vi "Main.vi"() -> ()   [LabVIEW 2012]
uses:
  ChannelStateControl.ctl
  <vilib>/Utility/error.llb/DialogType.ctl
  Imaging Pulse Control/Examples/Support/Channel Parameters.ctl
  Imaging Pulse Control/Examples/Support/System Parameters.ctl
  <vilib>/UeiDaq/UeiDaqCreateDOSession.vi
  <vilib>/UeiDaq/UeiDaqConfigureTimingForSimpleIO.vi
  <vilib>/ULx/Create Channel.llb/ULx Create Channel (AO-Voltage-Basic).vi
  <vilib>/ULx/Write.llb/ULx Write (Analog 1D DBL NChan 1Samp).vi
  <vilib>/UeiDaq/UeiDaqWriteDigitalDataUInt16.vi
  <vilib>/UeiDaq/UeiDaqWriteOneDigitalScanUInt16.vi
  <resource>/objmgr/UeiDaq.rc
  Imaging Pulse Control/Quantum Composers 9000 Series.lvlib
  IPG Pulse Control/Agilent 33XXX Series.lvlib
  Agilent ESG Series/Agilent ESG Series.lvlib
panel:
  in  "Composer Write":bool
  in  "VISA session":refnum<visa-resource-name>
  in  "error in (no error)":errorcluster {"code" format="%.0x"}
  out "error out":errorcluster {"code" format="%.0x"}
  in  "Frequency (MHz)":dbl=224.0 format="%.11f"
  in  "Amplitude (dBm)":dbl=7.0 format="%.2f"
  in  "Output Enable":bool=TRUE
  out "Offset":dbl
  out "Amplitude":dbl
  in  "Maximum Voltage":dbl=10.0
  in  "Initial Voltage":dbl=2.0
  in  "Final Voltage":dbl=4.0
  out "Frequency":dbl=0.4838
  in  "Trigger Source (0: Internal)":u16(ring)=1 items=["Internal", "External", "Software (bus)"]
  in  "Enable Burst":bool=TRUE
  in  "Burst Mode (0: Triggered)":u16(ring) items=["Triggered", "Gated"]
  out "Simulated WaveForm":dbl[](graph)
  out "Total Time  (<16000)":i32
  in  "Final Keep Time":i32=100
  in  "Fall Down Time":i32=1000
  in  "Rise Up Time":i32=15
  in  "Pulse Width":i32=100
  in  "Inintial Voltage Time":i32=1
  in  "IPG Controller (Agilent 33210A)":refnum<visa-resource-name>
  in  "Arbitrary Waveform Name":string="ARB1"
  in  "Run IPG Laser Control":bool
  in  "Normal Stop":bool
  in  "Voltage (V)":dbl[](array[numeric])
  in  "Initial States(Adjustable)":u16[](array[numeric])=[0, 0, 0, 0, 0, 0, 0, 0, 0, 0, 0, 0, 0, 0, 0, 0, 0, 0, 0, 0] caption="Initial States"
  in  "DIO Groups":T1[](array[typedef])
  out "Quantum Composer Command":string[](array[string])
  in  "Sys Period (s)":dbl=0.15
  out "Composer Ready?":bool
  out "Main Loop Stopped?":bool
  in  "Quantum Composer Resource":refnum<visa-resource-name>
  in  "Run/Stop":bool caption="stop"
  in  "Exit":bool
  out "Running 2":bool
  in  "Maximum Value":dbl=5.5 format="%0.2f"
  in  "Minimum Value":dbl format="%0.2f"
  out "Status Indicator":bool[][](array[boolean])
  out "Total Step":u64
  in  "Original Timing Signal (adjustable)":i16[][](array[numeric])=[[0, 0, 0, 0, 0, 0, 0, 0, 0, 0, 0, 0, 0, 0, 0, 0, 0, 0, 0, 0]] format="%b"
  out "Running":bool
  in  "DIO Port":string="pwrdaq://Dev0/Do0:2"
  in  "stop":bool
  out "Loop Count":i32
  in  "Loop":bool
  out "Parsed File Location":path
  in  "All Low":bool
  in  "Run":bool
  in  "Timing Array (Adjustable)":i32[](array[numeric])=[0, 0, 0, 0, 0, 0, 0, 0, 0, 0, 0, 0, 0, 0, 0, 0, 0, 0, 0, 0] caption="Timing Array (Time Duration for each signal)"
  out "Modified Timing Signal":u16[][](array[numeric]) caption="Modified Timing Signal (after adjustment from I/O channel panel)" format="%b"
  in  "Compile":bool
  out "Channel Names":string[](array[string])
  in  "Channel Number (Adjustable)":u16=48
  in  "Load":bool
  in  "Timing File":path
  in  "Perl Parser":path=path "C:/Labview/Parser File/parse-timing.pl"
  # "MCCDAQ Control"
  # "(Use Do0:5 for DIO0-DIO5, 6ch,  Do0;5 for DIO0 and DIO5, 2ch)"
  # "Control Panel"
  # "(pwrdaq://Dev0 for real I/O; simu://Dev2 for simulated DAQ card)"
  # "1"
  # "2"
  # "3"
  # "4"
  # "5"
  # "6"
  # "7"
  # "8"
  # "9"
  # "10"
  # "11"
  # "12"
  # "13"
  # "14"
  # "15"
  # "16"
  # "Quantum Composer Control"
  # "Read me: (Very Important!!!!!!!!!)\n1. This Labview is used to control the IPG laser output power, When you edit this programme make sure the IPG laser is off.\n2. follow the steps, First is the visa address setting; Second is the pulse edit; Third is the output checking; Forth is the trigger set .\n3. The maximum input voltage is 10V, the minmum value is 1V. The total input time must smaller than 16000ms and larger than 8 ms."
  # "Group1"
  # "Group2"
  # "Group3"
  # "IPG Modulation Control"
  # "Offset Locking Control"
  # "Group4"
  # "Group5"
  # "Group6"
  # "(Currently, When \"STOP Loop\" is pressed, the status remain in the final state, when Stop Program or ER stop is pressed, all channels will be set as \"low\")"
  # "Status Panel"
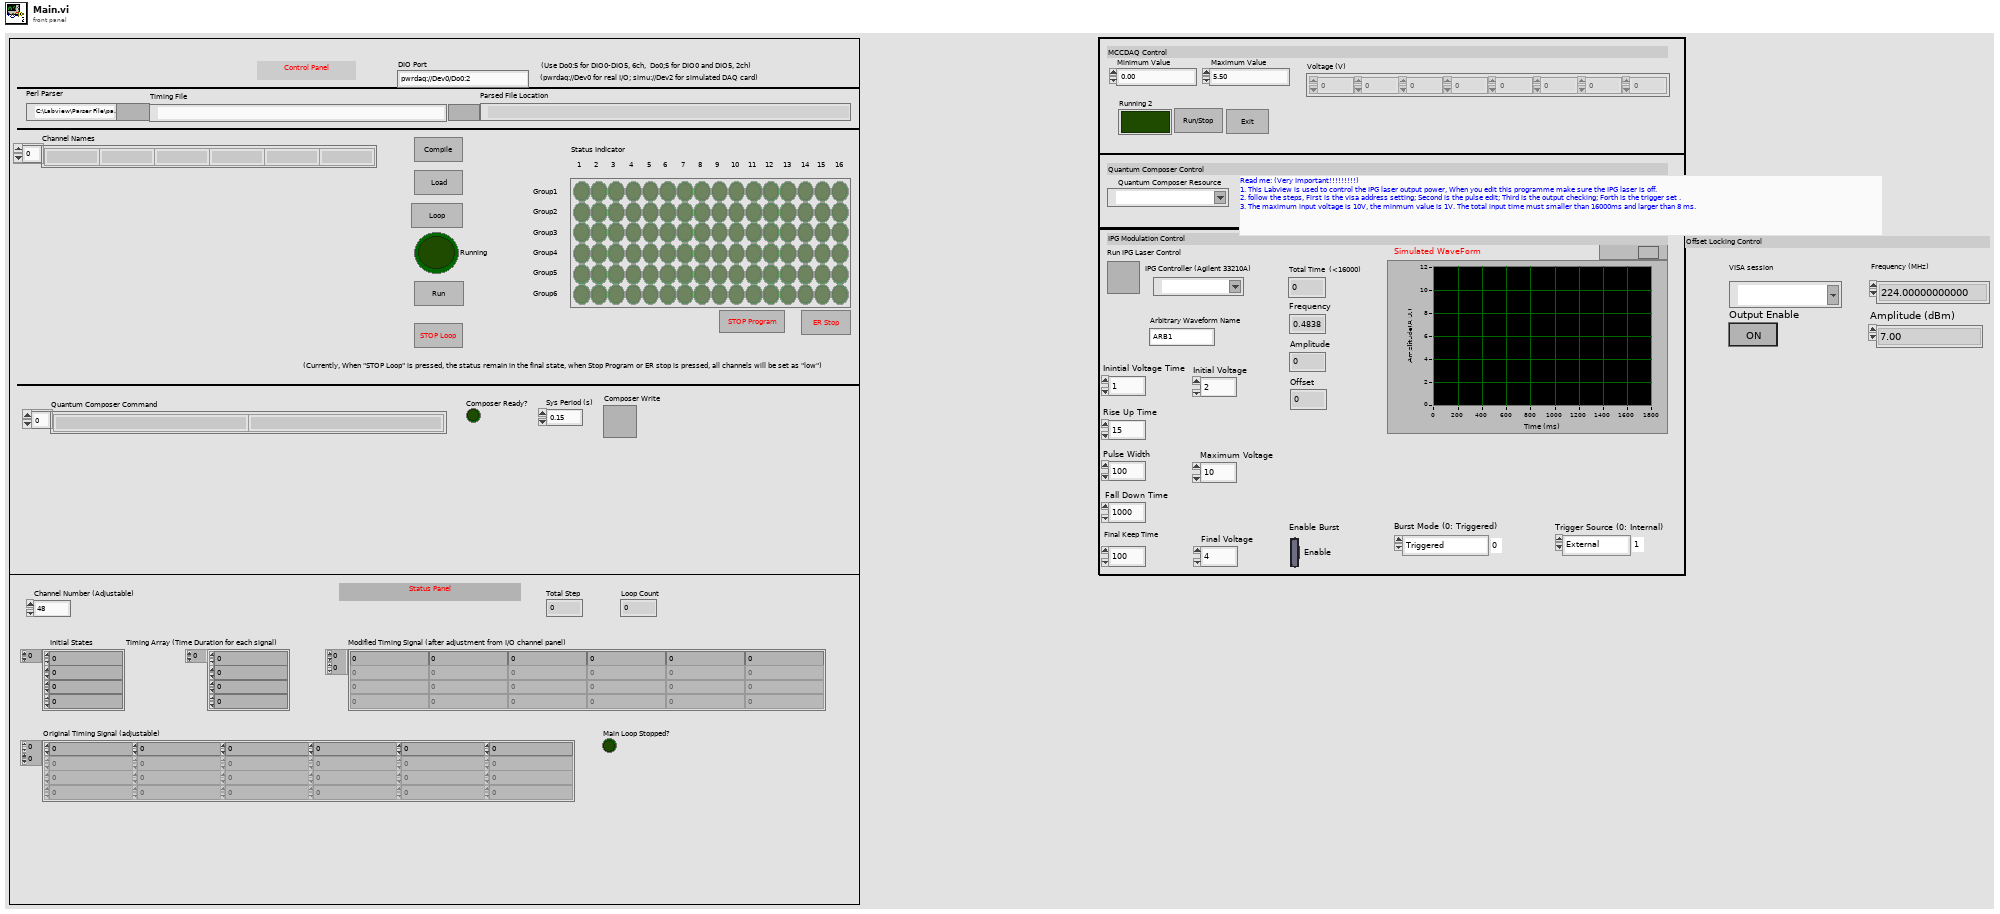
[diagram p1: front panel]
types:
  T1 = typedef "ChannelStateControl.ctl" = cluster{"Channel 1":u8, "Enable":bool, "Main Switch":u8, "Channel 2":u8, "Channel 9":u8, "Channel 10":u8, "Channel 11":u8, "Channel 3":u8, "Channel 4":u8, "Channel 12":u8, "Channel 5":u8, "Channel 13":u8, "Channel 6":u8, "Channel 14":u8, "Channel 7":u8, "Channel 15":u8, "Channel 8":u8, "Channel 16":u8}
  T2 = typedef "Channel Parameters.ctl" = cluster{"Channel":i32, "Chan State":bool, "Chan Sync Source":i32, "Chan Gate Logic":enum16{"Disabled", "Low", "High"}, "Chan Mode":enum16{"Normal", "Single", "Burst", "Duty Cycle"}, "Chan Wait #":i32, "Chan Delay":dbl, "Chan Width":dbl, "Chan Burst #":i32, "Chan DC On":i32, "Chan DC Off":i32, "Chan Polarity":bool, "Chan MUX Value":i32, "Chan Level Out":enum16{"TTL", "Adjustable", "35 Volt", "Optical"}, "Chan Lev Adjust":dbl, "Chan Gate Mode":enum16{"Disabled", "Pulse Inhibit", "Output Inhibit"}}
  T3 = typedef "DialogType.ctl" = u16
  T4 = typedef "System Parameters.ctl" = cluster{"Sys Period":dbl, "Sys Mode":enum16{"Normal", "Single", "Burst", "Duty Cycle"}, "Sys Burst #":i32, "Sys DC On":i32, "Sys DC Off":i32, "Sys State":bool, "Sys Gate":bool, "Sys Trig Edge":bool, "Sys Ext Mode":enum16{"Disabled", "Triggered", "Gated", "Triggered & Gated"}, "Sys Trig Lev":dbl, "Sys Gate Lev ":dbl, "Sys Gate Mode":enum16{"Disabled", "Pulse Inhibit", "Output Inhibit", "Channel"}}
  T5 = cluster{"Baud Rate":u32, "Parity":u16, "Data Bits":u16, "Flow Control":u16}
  T6 = enum16{"dBm", "dBuV", "dBuVemf", "mV", "uV", "mVemf", "uVemf"}
  T7 = enum16{"SINE", "TRIANGLE", "SQUARE", "RAMP", "NOISE", "DUAL SINE", "SWEPT SINE"}
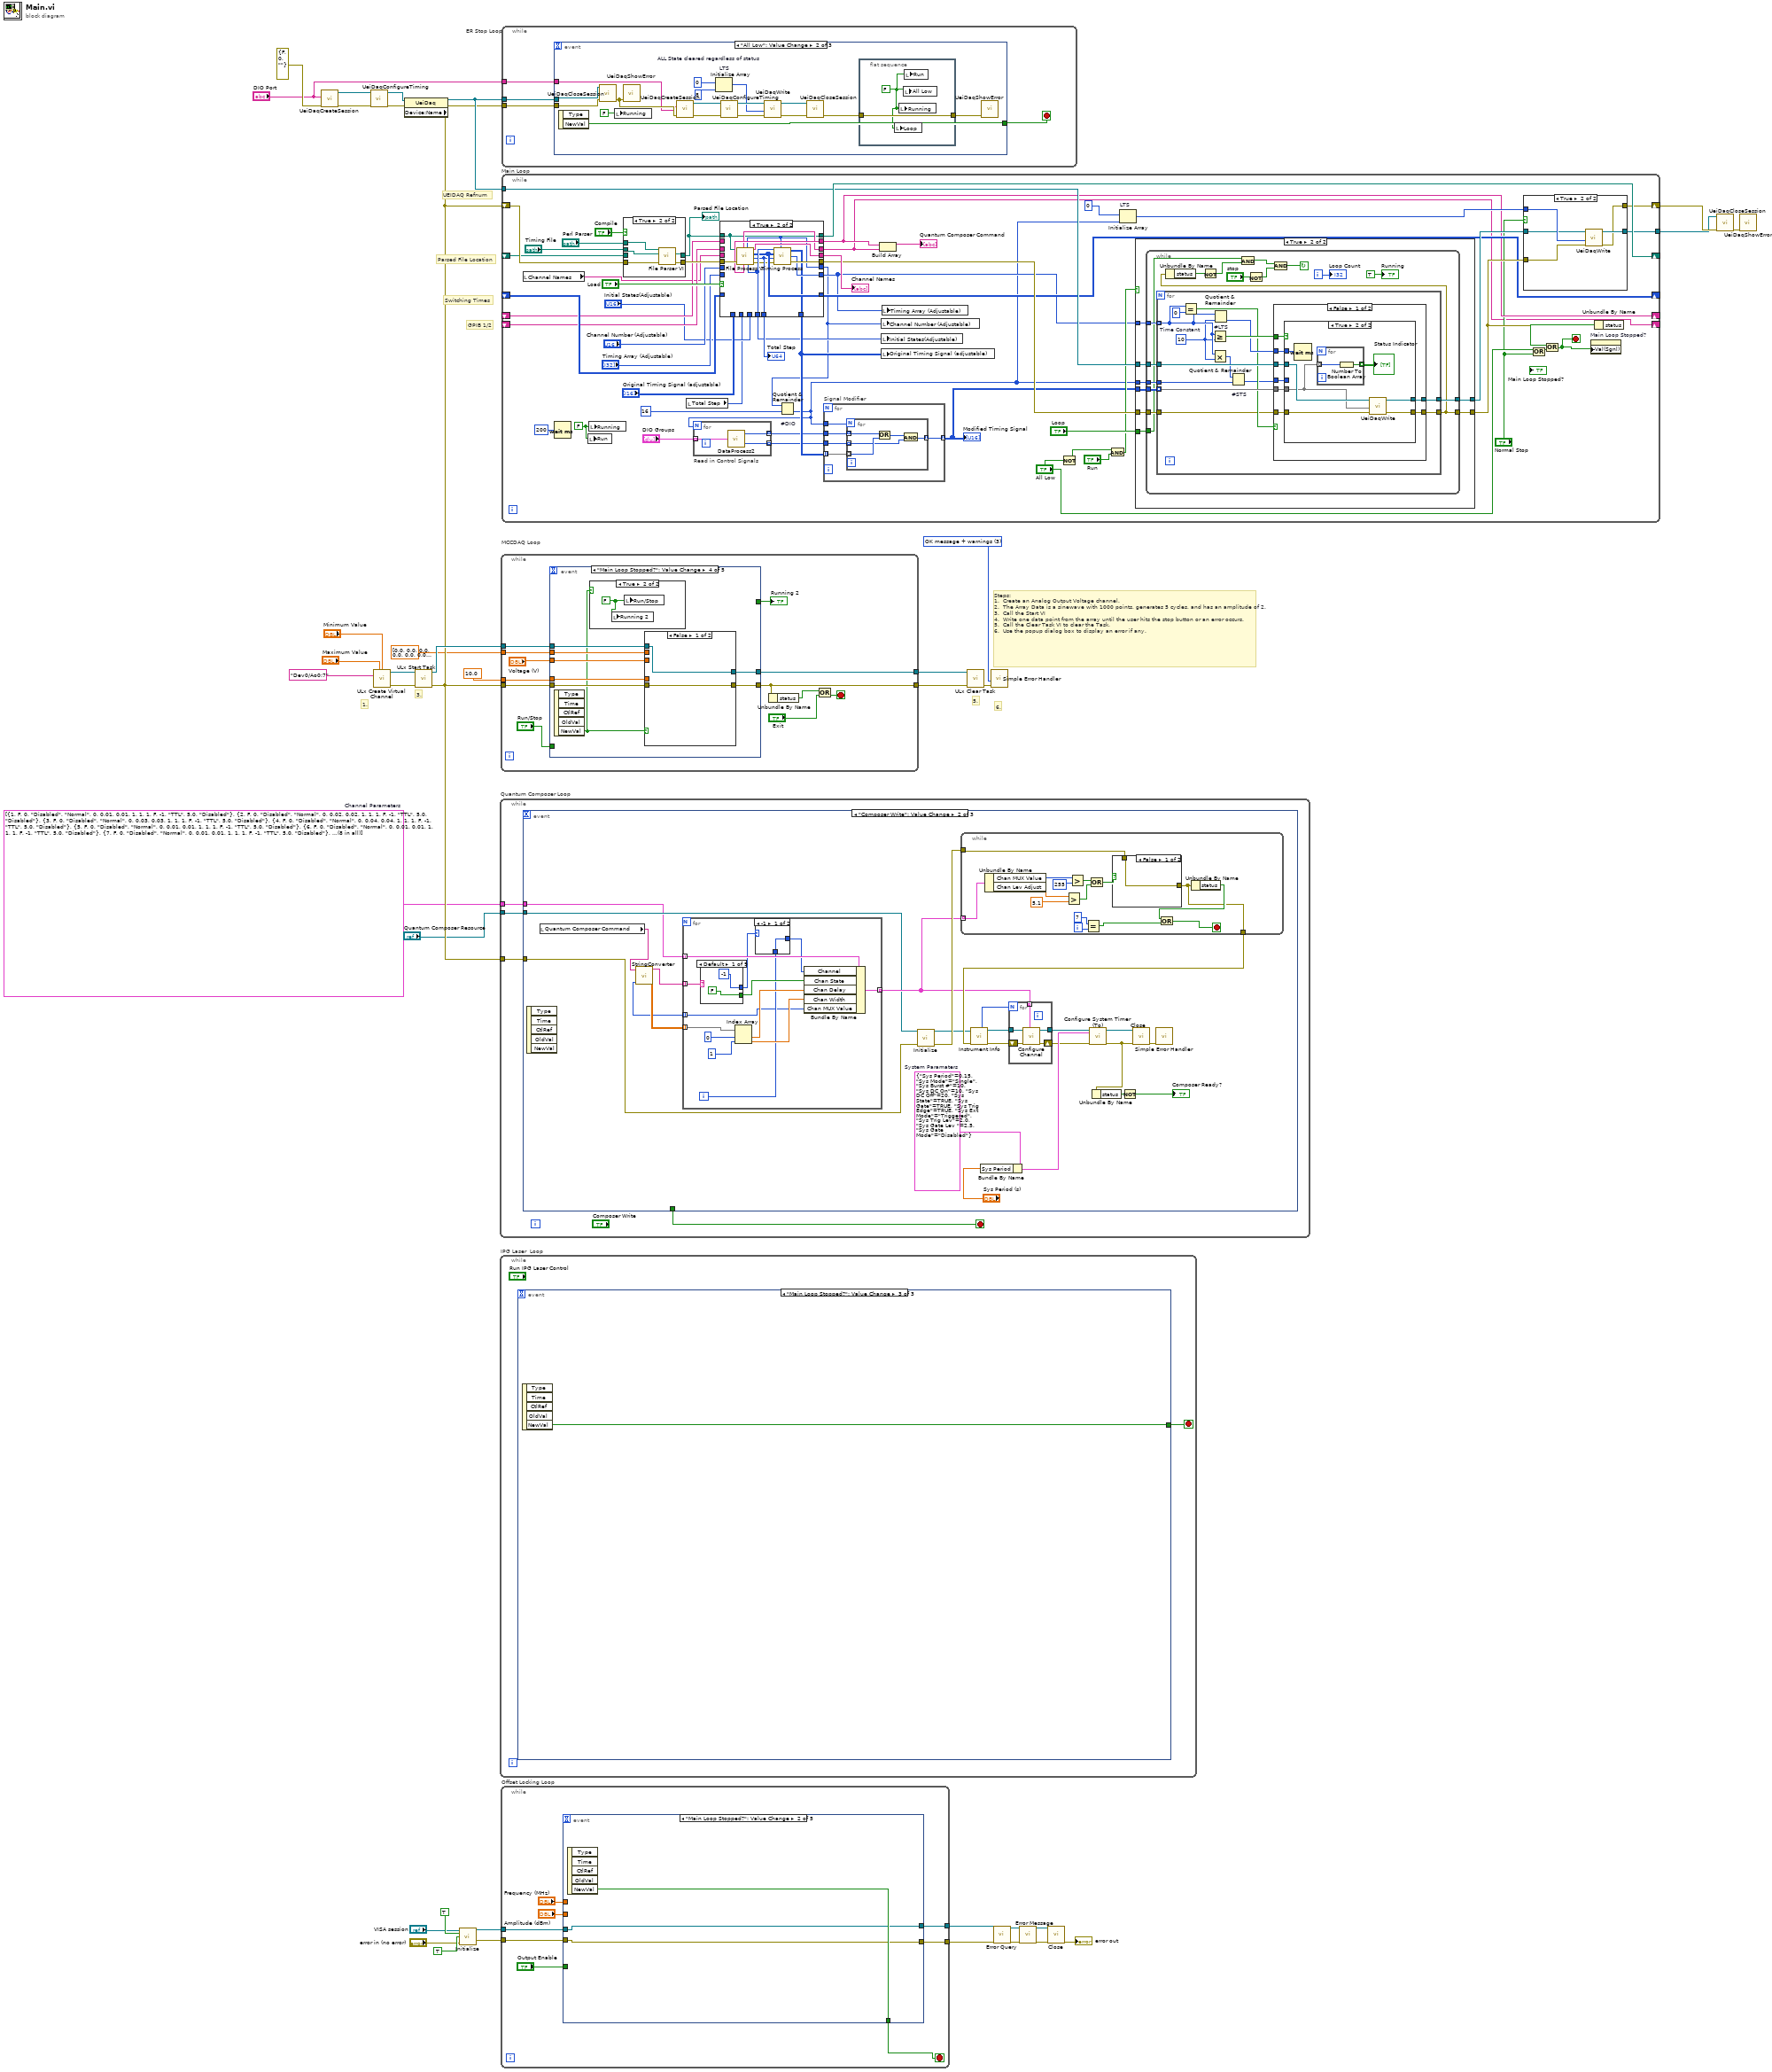
[diagram p0: block diagram]
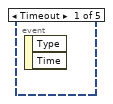
[diagram p2: hidden frame]
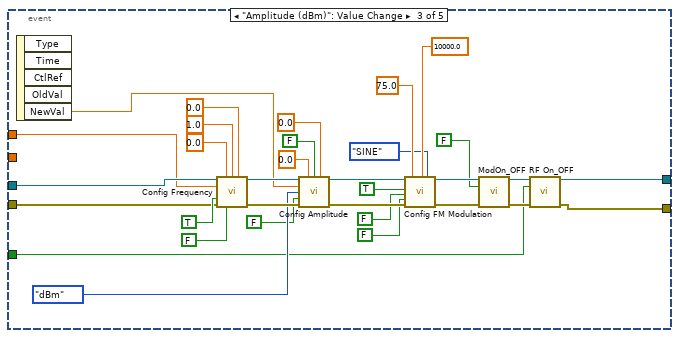
[diagram p3: hidden frame]
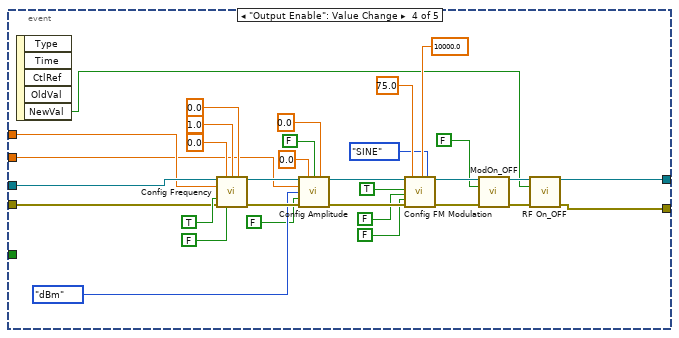
[diagram p4: hidden frame]
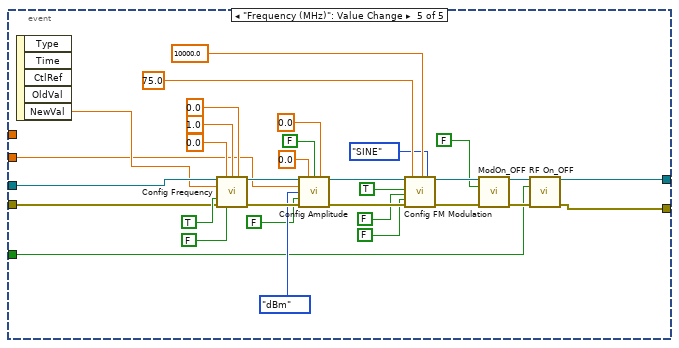
[diagram p5: hidden frame]
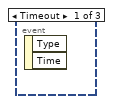
[diagram p6: hidden frame]
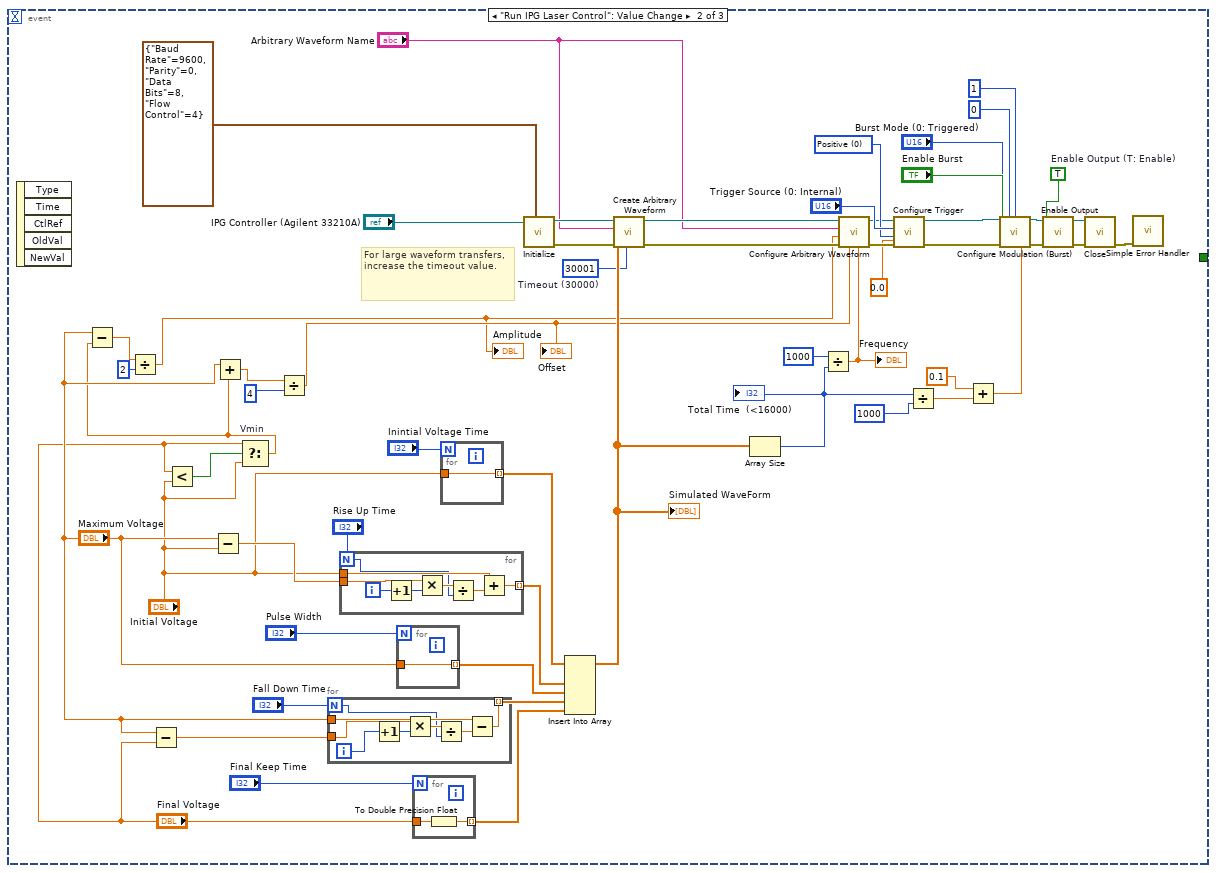
[diagram p7: hidden frame]
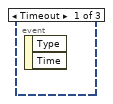
[diagram p8: hidden frame]
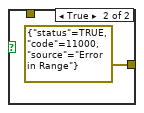
[diagram p9: hidden frame]
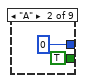
[diagram p11: hidden frame]
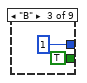
[diagram p12: hidden frame]
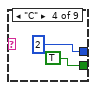
[diagram p13: hidden frame]
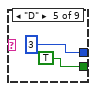
[diagram p14: hidden frame]
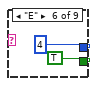
[diagram p15: hidden frame]
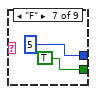
[diagram p16: hidden frame]
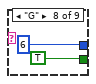
[diagram p17: hidden frame]
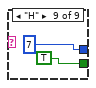
[diagram p18: hidden frame]
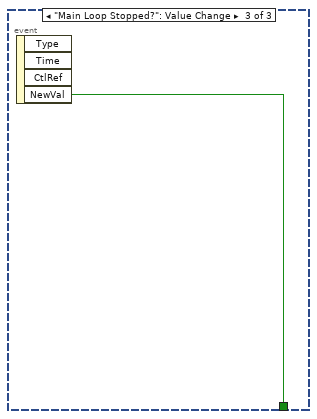
[diagram p19: hidden frame]
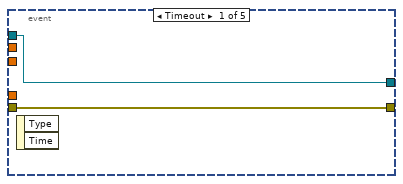
[diagram p20: hidden frame]
diagram:
  w1 = T2[] [{"Channel"=1, "Chan State"=FALSE, "Chan Sync Source"=0, "Chan Gate Logic"=enum."Disabled", "Chan Mode"=enum."Normal", "Chan Wait #"=0, "Chan Delay"=0.01, "Chan Width"=0.01, "Chan Burst #"=1, "Chan DC On"=1, "Chan DC Off"=1, "Chan Polarity"=FALSE, "Chan MUX Value"=-1, "Chan Level Out"=enum."TTL", "Chan Lev Adjust"=5.0, "Chan Gate Mode"=enum."Disabled"}, {"Channel"=2, "Chan State"=FALSE, "Chan Sync Source"=0, "Chan Gate Logic"=enum."Disabled", "Chan Mode"=enum."Normal", "Chan Wait #"=0, "Chan Delay"=0.02, "Chan Width"=0.02, "Chan Burst #"=1, "Chan DC On"=1, "Chan DC Off"=1, "Chan Polarity"=FALSE, "Chan MUX Value"=-1, "Chan Level Out"=enum."TTL", "Chan Lev Adjust"=5.0, "Chan Gate Mode"=enum."Disabled"}, {"Channel"=3, "Chan State"=FALSE, "Chan Sync Source"=0, "Chan Gate Logic"=enum."Disabled", "Chan Mode"=enum."Normal", "Chan Wait #"=0, "Chan Delay"=0.03, "Chan Width"=0.03, "Chan Burst #"=1, "Chan DC On"=1, "Chan DC Off"=1, "Chan Polarity"=FALSE, "Chan MUX Value"=-1, "Chan Level Out"=enum."TTL", "Chan Lev Adjust"=5.0, "Chan Gate Mode"=enum."Disabled"}, {"Channel"=4, "Chan State"=FALSE, "Chan Sync Source"=0, "Chan Gate Logic"=enum."Disabled", "Chan Mode"=enum."Normal", "Chan Wait #"=0, "Chan Delay"=0.04, "Chan Width"=0.04, "Chan Burst #"=1, "Chan DC On"=1, "Chan DC Off"=1, "Chan Polarity"=FALSE, "Chan MUX Value"=-1, "Chan Level Out"=enum."TTL", "Chan Lev Adjust"=5.0, "Chan Gate Mode"=enum."Disabled"}, {"Channel"=5, "Chan State"=FALSE, "Chan Sync Source"=0, "Chan Gate Logic"=enum."Disabled", "Chan Mode"=enum."Normal", "Chan Wait #"=0, "Chan Delay"=0.01, "Chan Width"=0.01, "Chan Burst #"=1, "Chan DC On"=1, "Chan DC Off"=1, "Chan Polarity"=FALSE, "Chan MUX Value"=-1, "Chan Level Out"=enum."TTL", "Chan Lev Adjust"=5.0, "Chan Gate Mode"=enum."Disabled"}, {"Channel"=6, "Chan State"=FALSE, "Chan Sync Source"=0, "Chan Gate Logic"=enum."Disabled", "Chan Mode"=enum."Normal", "Chan Wait #"=0, "Chan Delay"=0.01, "Chan Width"=0.01, "Chan Burst #"=1, "Chan DC On"=1, "Chan DC Off"=1, "Chan Polarity"=FALSE, "Chan MUX Value"=-1, "Chan Level Out"=enum."TTL", "Chan Lev Adjust"=5.0, "Chan Gate Mode"=enum."Disabled"}, {"Channel"=7, "Chan State"=FALSE, "Chan Sync Source"=0, "Chan Gate Logic"=enum."Disabled", "Chan Mode"=enum."Normal", "Chan Wait #"=0, "Chan Delay"=0.01, "Chan Width"=0.01, "Chan Burst #"=1, "Chan DC On"=1, "Chan DC Off"=1, "Chan Polarity"=FALSE, "Chan MUX Value"=-1, "Chan Level Out"=enum."TTL", "Chan Lev Adjust"=5.0, "Chan Gate Mode"=enum."Disabled"}, {"Channel"=8, "Chan State"=FALSE, "Chan Sync Source"=0, "Chan Gate Logic"=enum."Disabled", "Chan Mode"=enum."Normal", "Chan Wait #"=0, "Chan Delay"=0.01, "Chan Width"=0.01, "Chan Burst #"=1, "Chan DC On"=1, "Chan DC Off"=1, "Chan Polarity"=FALSE, "Chan MUX Value"=-1, "Chan Level Out"=enum."TTL", "Chan Lev Adjust"=5.0, "Chan Gate Mode"=enum."Disabled"}]  # Channel Parameters
  w28 = T3 3 items=["no dialog", "OK message", "continue or stop message", "OK message + warnings", "continue/stop + warnings"] ("type of dialog (OK msg:1)")
  # "UEIDAQ Refnum"
  # "GPIB 1/2"
  # "Switching Times"
  # "Parsed File Location"
  # "6."
  # "5."
  # "Steps: \n1.  Create an Analog Output Voltage channel.\n2.  The Array Data is a sinewave with 1000 points, generates 5 cycles, and has an amplitude of 2.\n3.  Call the Start VI\n4.  Write one data point from the array until the user hits the stop button or an error occurs. \n5.  Call the Clear Task VI to clear the Task.\n6.  Use the popup dialog box to display an error if any."
  # "3."
  # "1."
  n1 = call-poly <vilib>:"UeiDaqCreateSession.vi"("error in (no error)"=errorcluster {"status"=FALSE, "code"=0, "source"=""} ("error constant"), "Resource"="DIO Port") -> ("error out"=w38:errorcluster, "UeiDaq Refnum Out"=w39:refnum<k20>)  [unwired: 8 in]
  n2 = call-poly <vilib>:"UeiDaqConfigureTiming.vi"("error in (no error)"=w38, "UeiDaq Refnum In"=w39) -> ("error out"=w36:errorcluster, "UeiDaq Refnum Out"=w37:refnum<k20>)  [unwired: 8 in]
  n3 = property class="UeiDaq" props=["Device:Name"](reference=w37, error in=w36) -> (reference out=w34:refnum<k20>, error out=w21:errorcluster)  [unwired: 1 out]
  n4 = call-poly <vilib>:"ULx Create Virtual Channel.vi"("maximum value"="Maximum Value", "minimum value"="Minimum Value", "physical channels"="Dev0/Ao0:7", "error in"=w21) -> ("task out"=w27:refnum<k24>, "error out"=w26:errorcluster)  [unwired: 10 in]
  n5 = call <vilib>:"ULx Start Task.vi"("task in"=w27, "error in"=w26) -> ("task out"=w29:refnum<k24>, "error out"=w31:errorcluster)  [unwired: 12 in]
  n6 = call "Initialize.vi"("VISA Resource Name"="VISA session", "ID Query? (T: Yes)"=TRUE, "Reset? (T: Yes)"=TRUE, "error in (no error)"="error in (no error)") -> ("VISA Resource Name Out"=w4:refnum<visa-resource-name>, "error out"=w3:errorcluster)  [unwired: 10 in]
  n7 = while "Quantum Composer Loop" {
    tunnel: "Quantum Composer Resource" -> [w42]
    tunnel: w21 -> [w43]
    tunnel: w1 -> [w40]
    stop <- w41 stop-if-true
    n8 = event shown="[1] \"Composer Write\": Value Change" {
      selector: _ -> [_ _ _]
      dyn-events: _ -> [_ _ _]
      timeout: _ -> [_ _ _]
      tunnel: w43 -> [_ w45 _]
      tunnel: w42 -> [_ w47 _]
      tunnel: w40 -> [_ w46 _]
      tunnel: [_ _ w123] -> w41
      event Timeout {
        n9 = event-data() -> ()  [unwired: 1 in, 2 out]
      }
      event "Composer Write": Value Change {
        w57 = T4 {"Sys Period"=0.15, "Sys Mode"=enum."Single", "Sys Burst #"=10, "Sys DC On"=10, "Sys DC Off"=20, "Sys State"=TRUE, "Sys Gate"=TRUE, "Sys Trig Edge"=TRUE, "Sys Ext Mode"=enum."Triggered", "Sys Trig Lev"=2.0, "Sys Gate Lev "=2.5, "Sys Gate Mode"=enum."Disabled"}  # System Paramaters
        n10 = event-data() -> ()  [unwired: 1 in, 5 out]
        n11 = local read "Quantum Composer Command"() -> (w44:string[])
        n12 = call "StringConverter.vi"("Composer Command"=w44) -> ("Internal Channel Delay and Width"=w63:dbl[][], "Internal Channel Name"=w64:string[], "Mux Value"=w62:i32[])  [unwired: 8 in]
        n13 = for {
          tunnel: w46 -> [w102] mode=indexing
          tunnel: w64 -> [w96] mode=indexing
          tunnel: w63 -> [w100] mode=indexing
          tunnel: [w91] -> w49 mode=indexing
          tunnel: w62 -> [w90] mode=indexing
          i -> [w92]
          n14 = case shown="Default" w96 {
            tunnel: [-1 0 1 2 3 4 5 6 7] -> w94
            tunnel: [FALSE TRUE TRUE TRUE TRUE TRUE TRUE TRUE TRUE] -> w95
            frame Default {
            }
            frame "A" {
            }
            frame "B" {
            }
            frame "C" {
            }
            frame "D" {
            }
            frame "E" {
            }
            frame "F" {
            }
            frame "G" {
            }
            frame "H" {
            }
          }
          n15 = Index Array(array=w100, index #1=0, index #2=1) -> (element #1=w101:dbl, element #2=w97:dbl)
          n16 = case shown="-1" w94 {
            selector: w94 -> [_ w104]
            tunnel: [w103 w104] -> w93
            tunnel: w92 -> [w103 _]
            frame -1 {
            }
            frame Default {
            }
          }
          n17 = Bundle By Name(cluster=w102, "Channel"=w93, "Chan State"=w95, "Chan Delay"=w101, "Chan Width"=w97, "Chan MUX Value"=w90) -> (w91:T2)
        }
        n18 = call "Initialize.vi"("error in (no error)"=w45, "VISA resource name"=w47) -> ("error out"=w60:errorcluster, "VISA resource name out"=w48:refnum<visa-resource-name>)  [unwired: 8 in]
        n19 = while {
          tunnel: w49 -> [w87] mode=indexing
          tunnel: [w73] -> w61
          tunnel: w60 -> [w74]
          i -> [w85]
          stop <- w75 stop-if-true
          n20 = Unbundle By Name(w87) -> ("Chan MUX Value"=w80:i32, "Chan Lev Adjust"=w83:dbl)
          n21 = Greater?(x=w83, y=5.1) -> (0:w81:bool)
          n22 = Greater?(x=w80, y=255) -> (0:w78:bool)
          n23 = Equal?(x=7, y=w85) -> (x = y?=w77:bool)
          n24 = Or(x=w78, y=w81) -> (x .or. y?=w82:bool)
          n25 = case shown="False" w82 {
            tunnel: [w88 errorcluster {"status"=TRUE, "code"=11000, "source"="Error in Range"} ("error constant")] -> w73
            tunnel: w74 -> [w88 _]
            frame False {
            }
            frame True {
            }
          }
          n26 = Unbundle By Name(w73) -> ("status"=w76:bool)
          n27 = Or(x=w76, y=w77) -> (x .or. y?=w75:bool)
        }
        n28 = call "Instrument Info.vi"("error in (no error)"=w61, "VISA resource name"=w48) -> ("error out"=w51:errorcluster, "VISA resource name out"=w50:refnum<visa-resource-name>, "Channels"=w52:i32)  [unwired: 6 in, 1 out]
        n29 = Bundle By Name(cluster=w57, "Sys Period"="Sys Period (s)") -> (w59:T4)
        n30 = for {
          N: w52 -> [_]
          tunnel: [w72] -> w53
          tunnel: w49 -> [w71] mode=indexing
          tunnel: w50 -> [w70]
          shift-right: [w69] -> w54
          shift-left: w51 -> [w68]
          n31 = call "Configure Channel.vi"("Chan Parameters"=w71, "error in (no error)"=w68, "VISA resource name"=w70) -> ("error out"=w69:errorcluster, "VISA resource name out"=w72:refnum<visa-resource-name>)  [unwired: 7 in]
        }
        n32 = call "Configure System Timer (To).vi"("System Parameters"=w59, "error in (no error)"=w54, "VISA resource name"=w53) -> ("error out"=w67:errorcluster, "VISA resource name out"=w66:refnum<visa-resource-name>)  [unwired: 7 in]
        n33 = Unbundle By Name(w67) -> ("status"=w55:bool)
        n34 = Not(x=w55) -> (.not. x?=→"Composer Ready?":bool)
        n35 = call "Close.vi"("error in (no error)"=w67, "VISA resource name"=w66) -> ("error out"=w65:errorcluster)  [unwired: 9 in]
        n36 = call <vilib>:"Simple Error Handler.vi"("error in (no error)"=w65) -> ()  [unwired: 4 in, 5 out]
      }
      event "Main Loop Stopped?": Value Change {
        n37 = event-data() -> ("NewVal"=w123:bool)  [unwired: 1 in, 3 out]
      }
    }
  }
  n38 = while "IPG Laser  Loop" {
    stop <- w124 stop-if-true
    n39 = event shown="[2] \"Main Loop Stopped?\": Value Change" {
      selector: _ -> [_ _ _]
      dyn-events: _ -> [_ _ _]
      timeout: _ -> [_ _ _]
      tunnel: [_ _ w201] -> w124
      event Timeout {
        n40 = event-data() -> ()  [unwired: 1 in, 2 out]
      }
      event "Run IPG Laser Control": Value Change {
        w164 = u16 0 items=["Positive", "Negative"] ("Slope (0: Positive)")
        w140 = u32 30001  # Timeout (30000)
        w177 = TRUE  # Enable Output (T: Enable)
        # "For large waveform transfers, increase the timeout value."
        n41 = event-data() -> ()  [unwired: 1 in, 5 out]
        n42 = Subtract(x="Maximum Voltage", y="Final Voltage") -> (x-y=w136:dbl)
        n43 = Less?(x="Final Voltage", y="Initial Voltage") -> (x < y?=w135:bool)
        n44 = Subtract(x="Maximum Voltage", y="Initial Voltage") -> (x-y=w138:dbl)
        n45 = Select "Vmin"(t="Final Voltage", s=w135, f="Initial Voltage") -> (s? t:f=w131:dbl)
        n46 = Subtract(x="Maximum Voltage", y=w131) -> (x-y=w134:dbl)
        n47 = Divide(x=w134, y=2) -> (x/y=w125:dbl)
        "Amplitude" <- w125
        n48 = Add(x="Maximum Voltage", y=w131) -> (x+y=w130:dbl)
        n49 = Divide(x=w130, y=4) -> (x/y=w128:dbl)
        "Offset" <- w128
        n50 = for {
          N: "Fall Down Time" -> [w184]
          tunnel: [w189] -> w168 mode=indexing
          tunnel: w136 -> [w186]
          tunnel: "Maximum Voltage" -> [w185]
          i -> [w188]
          n51 = Increment(x=w188) -> (x+1=w187:i32)
          n52 = Multiply(x=w186, y=w187) -> (x*y=w191:dbl)
          n53 = Divide(x=w191, y=w184) -> (x/y=w190:dbl)
          n54 = Subtract(x=w185, y=w190) -> (x-y=w189:dbl)
        }
        n55 = for {
          N: "Rise Up Time" -> [w194]
          tunnel: [w199] -> w172 mode=indexing
          tunnel: "Initial Voltage" -> [w198]
          tunnel: w138 -> [w196]
          i -> [w200]
          n56 = Increment(x=w200) -> (x+1=w197:i32)
          n57 = Multiply(x=w196, y=w197) -> (x*y=w195:dbl)
          n58 = Divide(x=w195, y=w194) -> (x/y=w193:dbl)
          n59 = Add(x=w198, y=w193) -> (x+y=w199:dbl)
        }
        n60 = for {
          N: "Pulse Width" -> [_]
          tunnel: [w192] -> w169 mode=indexing
          tunnel: "Maximum Voltage" -> [w192]
        }
        n61 = for {
          N: "Final Keep Time" -> [_]
          tunnel: [w181] -> w166 mode=indexing
          tunnel: "Final Voltage" -> [w182]
          n62 = To Double Precision Float(number=w182) -> (double precision float=w181:dbl)
        }
        n63 = for {
          N: "Inintial Voltage Time" -> [_]
          tunnel: [w183] -> w170 mode=indexing
          tunnel: "Initial Voltage" -> [w183]
        }
        n64 = call "Initialize.vi"("Serial Configuration"=T5 {"Baud Rate"=9600, "Parity"=0, "Data Bits"=8, "Flow Control"=4}, "VISA resource name"="IPG Controller (Agilent 33210A)") -> ("error out"=w142:errorcluster, "VISA resource name out"=w145:refnum<visa-resource-name>)  [unwired: 8 in]
        n65 = Insert Into Array(array=w170, new element #1=w172, new element #2=w169, new element #3=w168, new element #4=w166) -> (w143:dbl[])  [unwired: 1 in]
        "Simulated WaveForm" <- w143
        n66 = call "Create Arbitrary Waveform.vi"("Timeout (10000)"=w140, "error in (no error)"=w142, "Arbitrary Waveform Data"=w143, "Arbitrary Waveform Name (\"ARB1\")"="Arbitrary Waveform Name", "VISA resource name"=w145) -> ("error out"=w141:errorcluster, "VISA resource name out"=w144:refnum<visa-resource-name>)  [unwired: 5 in]
        n67 = Array Size(array=w143) -> (size(s)=w150:i32)
        "Total Time  (<16000)" <- w150
        n68 = Divide(x=1000, y=w150) -> (x/y=w151:dbl)
        "Frequency" <- w151
        n69 = call "Configure Arbitrary Waveform.vi"("Frequency (1000 Hz)"=w151, "Offset (0.00 V)"=w128, "error in (no error)"=w141, "Gain (1.0)"=w125, "Arbitrary Waveform Name (\"ARB1\")"="Arbitrary Waveform Name", "VISA resource name"=w144) -> ("error out"=w162:errorcluster, "VISA resource name out"=w163:refnum<visa-resource-name>)  [unwired: 4 in]
        n70 = call "Configure Trigger.vi"("Delay (0.0 s)"=0.0, "error in (no error)"=w162, "Slope (0: Positive)"=w164, "Trigger Source (0: Internal)"="Trigger Source (0: Internal)", "VISA resource name"=w163) -> ("error out"=w160:errorcluster, "VISA resource name out"=w161:refnum<visa-resource-name>)  [unwired: 5 in]
        n71 = Divide(x=w150, y=1000) -> (x/y=w148:dbl)
        n72 = Add(x=0.1, y=w148) -> (x+y=w146:dbl)
        n73 = call "Configure Modulation (Burst).vi"("VISA resource name"=w161, "Burst Phase (0 deg)"=0, "Burst Count (1)"=1, "Burst Period (1 s)"=w146, "Enable Burst Modulation (T: Enable)"="Enable Burst", "Burst Modulation Mode (0: Triggered)"="Burst Mode (0: Triggered)", "error in (no error)"=w160) -> ("VISA resource name out"=w159:refnum<visa-resource-name>, "error out"=w158:errorcluster)  [unwired: 7 in]
        n74 = call "Enable Output.vi"("error in (no error)"=w158, "Enable Output  (T: Enable)"=w177, "VISA resource name"=w159) -> ("error out"=w179:errorcluster, "VISA resource name out"=w178:refnum<visa-resource-name>)  [unwired: 7 in]
        n75 = call "Close.vi"("error in (no error)"=w179, "VISA resource name"=w178) -> ("error out"=w180:errorcluster)  [unwired: 9 in]
        n76 = call <vilib>:"Simple Error Handler.vi"("error in (no error)"=w180) -> ()  [unwired: 4 in, 5 out]
      }
      event "Main Loop Stopped?": Value Change {
        n77 = event-data() -> ("NewVal"=w201:bool)  [unwired: 1 in, 4 out]
      }
    }
  }
  n78 = while "MCCDAQ Loop" {
    tunnel: w31 -> [w212]
    tunnel: w29 -> [w213]
    tunnel: dbl[] [0.0, 0.0, 0.0, 0.0, 0.0, 0.0, 0.0, 0.0] -> [w209]
    tunnel: [w211] -> w24
    tunnel: [w208] -> w23
    tunnel: 10.0 ("timeout") -> [w210]
    stop <- w207 stop-if-true
    n79 = event shown="[3] \"Main Loop Stopped?\": Value Change" {
      selector: _ -> [_ _ _ _ _]
      dyn-events: _ -> [_ _ _ _ _]
      timeout: _ -> [_ _ _ _ _]
      tunnel: w213 -> [w215 w223 w243 w260 w277]
      tunnel: w212 -> [w214 w222 w242 w259 w276]
      tunnel: w210 -> [_ w221 w241 w258 w275]
      tunnel: "Voltage (V)" -> [_ w220 w240 w257 _]
      tunnel: [w215 w219 w239 w256 w274] -> w211
      tunnel: [w214 w218 w238 w255 w273] -> w208
      tunnel: w209 -> [_ w217 w237 w254 w272]
      tunnel: "Run/Stop" -> [_ _ _ _ w271]
      tunnel: [_ w216 _ _ _] -> w203
      event Timeout {
        n80 = event-data() -> ()  [unwired: 1 in, 2 out]
      }
      event "Run/Stop": Value Change {
        n81 = event-data() -> ("NewVal"=w216:bool)  [unwired: 1 in, 4 out]
        n82 = case shown="False" w216 {
          tunnel: w223 -> [w227 w235]
          tunnel: w222 -> [w226 w234]
          tunnel: w221 -> [w228 w233]
          tunnel: w220 -> [_ w232]
          tunnel: [w225 w231] -> w219
          tunnel: [w224 w230] -> w218
          tunnel: w217 -> [w229 _]
          frame False {
            n83 = call-poly <vilib>:"ULx Write.vi"("task in"=w227, "data"=w229, "timeout"=w228, "error in"=w226) -> ("task out"=w225:refnum<k24>, "error out"=w224:errorcluster)  [unwired: 9 in, 1 out]
          }
          frame True {
            n84 = call-poly <vilib>:"ULx Write.vi"("task in"=w235, "data"=w232, "timeout"=w233, "error in"=w234) -> ("task out"=w231:refnum<k24>, "error out"=w230:errorcluster)  [unwired: 9 in, 1 out]
          }
        }
      }
      event "Exit": Value Change {
        n85 = event-data() -> ("NewVal"=w236:bool)  [unwired: 1 in, 4 out]
        n86 = case shown="True" w236 {
          frame False {
          }
          frame True {
            w244 = FALSE
            n87 = local write "Running 2"(w244) -> ()
            n88 = local write "Run/Stop"(w244) -> ()
          }
        }
        n89 = case shown="True" w236 {
          tunnel: w243 -> [w246 w252]
          tunnel: w242 -> [w245 w251]
          tunnel: w241 -> [_ w250]
          tunnel: w240 -> [_ _]
          tunnel: [w246 w249] -> w239
          tunnel: [w245 w248] -> w238
          tunnel: w237 -> [_ w247]
          frame False {
          }
          frame True {
            n90 = call-poly <vilib>:"ULx Write.vi"("task in"=w252, "data"=w247, "timeout"=w250, "error in"=w251) -> ("task out"=w249:refnum<k24>, "error out"=w248:errorcluster)  [unwired: 9 in, 1 out]
          }
        }
      }
      event "Main Loop Stopped?": Value Change {
        n91 = event-data() -> ("NewVal"=w253:bool)  [unwired: 1 in, 4 out]
        n92 = case shown="True" w253 {
          frame False {
          }
          frame True {
            w261 = FALSE
            n93 = local write "Running 2"(w261) -> ()
            n94 = local write "Run/Stop"(w261) -> ()
          }
        }
        n95 = case shown="False" w253 {
          tunnel: w260 -> [w263 w269]
          tunnel: w259 -> [w262 w268]
          tunnel: w258 -> [_ w267]
          tunnel: w257 -> [_ _]
          tunnel: [w263 w266] -> w256
          tunnel: [w262 w265] -> w255
          tunnel: w254 -> [_ w264]
          frame False {
          }
          frame True {
            n96 = call-poly <vilib>:"ULx Write.vi"("task in"=w269, "data"=w264, "timeout"=w267, "error in"=w268) -> ("task out"=w266:refnum<k24>, "error out"=w265:errorcluster)  [unwired: 9 in, 1 out]
          }
        }
      }
      event "Voltage (V)": Value Change {
        n97 = event-data() -> ("NewVal"=w270:dbl[])  [unwired: 1 in, 4 out]
        n98 = case shown="True" w271 {
          tunnel: w277 -> [w281 w289]
          tunnel: w276 -> [w280 w288]
          tunnel: w275 -> [w282 w287]
          tunnel: w270 -> [_ w286]
          tunnel: [w279 w285] -> w274
          tunnel: [w278 w284] -> w273
          tunnel: w272 -> [w283 _]
          frame False {
            n99 = call-poly <vilib>:"ULx Write.vi"("task in"=w281, "data"=w283, "timeout"=w282, "error in"=w280) -> ("task out"=w279:refnum<k24>, "error out"=w278:errorcluster)  [unwired: 9 in, 1 out]
          }
          frame True {
            n100 = call-poly <vilib>:"ULx Write.vi"("task in"=w289, "data"=w286, "timeout"=w287, "error in"=w288) -> ("task out"=w285:refnum<k24>, "error out"=w284:errorcluster)  [unwired: 9 in, 1 out]
          }
        }
      }
    }
    "Running 2" <- w203
    n101 = Unbundle By Name(w208) -> ("status"=w206:bool)
    n102 = Or(x=w206, y="Exit") -> (x .or. y?=w207:bool)
  }
  n103 = while "Offset Locking Loop" {
    tunnel: [w297] -> w9
    tunnel: w4 -> [w296]
    tunnel: w3 -> [w295]
    tunnel: [w294] -> w2
    stop <- w292 stop-if-true
    n104 = event shown="[1] \"Main Loop Stopped?\": Value Change" {
      selector: _ -> [_ _ _ _ _]
      dyn-events: _ -> [_ _ _ _ _]
      timeout: _ -> [_ _ _ _ _]
      tunnel: [_ w298 w307 w339 w371] -> w297
      tunnel: w296 -> [_ w299 w306 w338 w370]
      tunnel: w295 -> [_ w298 w305 w337 w369]
      tunnel: "Output Enable" -> [_ _ w304 _ w366]
      tunnel: [_ w299 w303 w336 w365] -> w294
      tunnel: "Frequency (MHz)" -> [_ _ w301 w335 _]
      tunnel: [_ w300 _ _ _] -> w292
      tunnel: "Amplitude (dBm)" -> [_ _ _ w334 w367]
      event Timeout {
        n105 = event-data() -> ()  [unwired: 1 in, 2 out]
      }
      event "Main Loop Stopped?": Value Change {
        n106 = event-data() -> ("NewVal"=w300:bool)  [unwired: 1 in, 4 out]
      }
      event "Amplitude (dBm)": Value Change {
        n107 = event-data() -> ("NewVal"=w302:dbl)  [unwired: 1 in, 4 out]
        n108 = call "Config Frequency.vi"("VISA Resource Name"=w306, "Freq Offset (0.0)"=0.0, "Freq Multiplier (1.0)"=1.0, "Adjust Phase (0.0)"=0.0, "Frequency (1000.0)"=w301, "Freq Ref (T:ON)"=TRUE, "error in (no error)"=w305, "OptPhNoise (F:MD2 > 10khzOffset)"=FALSE) -> ("VISA Resource Name Out"=w332:refnum<visa-resource-name>, "error out"=w331:errorcluster)  [unwired: 6 in]
        n109 = call "Config Amplitude.vi"("VISA Resource Name"=w332, "Ampl Ref Set (0.00)"=0.0, "Ampl Ref (F:OFF)"=FALSE, "Ampl Offset (0.00)"=0.0, "Amplitude (-135.00)"=w302, "Unit (0:dBm)"=T6."dBm", "Atten Hold (F:OFF)"=FALSE, "error in (no error)"=w331) -> ("VISA Resource Name Out"=w330:refnum<visa-resource-name>, "error out"=w329:errorcluster)  [unwired: 6 in]
        n110 = call "Config FM Modulation.vi"("VISA Resource Name"=w330, "Status (T:ON)"=TRUE, "EXT Source Coupling (F:DC)"=FALSE, "FM Deviation Couple (F:OFF)"=FALSE, "error in (no error)"=w329, "FM Deviation (1.0)"=75.0 ("FM Deviation (75)"), "FM Rate (400.0)"=10000.0 ("FM Rate (10000)"), "FM Waveform (0:SINE)"=T7."SINE") -> ("VISA Resource Name Out"=w328:refnum<visa-resource-name>, "error out"=w327:errorcluster)  [unwired: 10 in]
        n111 = call "ModOn_OFF.vi"("VISA Resource Name"=w328, "Status (T:ON)"=FALSE, "error in (no error)"=w327) -> ("VISA Resource Name Out"=w326:refnum<visa-resource-name>, "error out"=w325:errorcluster)  [unwired: 11 in]
        n112 = call "RF On_OFF.vi"("VISA Resource Name"=w326, "Status (T:ON)"=w304, "error in (no error)"=w325) -> ("VISA Resource Name Out"=w303:refnum<visa-resource-name>, "error out"=w307:errorcluster)  [unwired: 11 in]
      }
      event "Output Enable": Value Change {
        n113 = event-data() -> ("NewVal"=w333:bool)  [unwired: 1 in, 4 out]
        n114 = call "Config Frequency.vi"("VISA Resource Name"=w338, "Freq Offset (0.0)"=0.0, "Freq Multiplier (1.0)"=1.0, "Adjust Phase (0.0)"=0.0, "Frequency (1000.0)"=w335, "Freq Ref (T:ON)"=TRUE, "error in (no error)"=w337, "OptPhNoise (F:MD2 > 10khzOffset)"=FALSE) -> ("VISA Resource Name Out"=w364:refnum<visa-resource-name>, "error out"=w363:errorcluster)  [unwired: 6 in]
        n115 = call "Config Amplitude.vi"("VISA Resource Name"=w364, "Ampl Ref Set (0.00)"=0.0, "Ampl Ref (F:OFF)"=FALSE, "Ampl Offset (0.00)"=0.0, "Amplitude (-135.00)"=w334, "Unit (0:dBm)"=T6."dBm", "Atten Hold (F:OFF)"=FALSE, "error in (no error)"=w363) -> ("VISA Resource Name Out"=w362:refnum<visa-resource-name>, "error out"=w361:errorcluster)  [unwired: 6 in]
        n116 = call "Config FM Modulation.vi"("VISA Resource Name"=w362, "Status (T:ON)"=TRUE, "EXT Source Coupling (F:DC)"=FALSE, "FM Deviation Couple (F:OFF)"=FALSE, "error in (no error)"=w361, "FM Deviation (1.0)"=75.0 ("FM Deviation (75)"), "FM Rate (400.0)"=10000.0 ("FM Rate (10000)"), "FM Waveform (0:SINE)"=T7."SINE") -> ("VISA Resource Name Out"=w360:refnum<visa-resource-name>, "error out"=w359:errorcluster)  [unwired: 10 in]
        n117 = call "ModOn_OFF.vi"("VISA Resource Name"=w360, "Status (T:ON)"=FALSE, "error in (no error)"=w359) -> ("VISA Resource Name Out"=w358:refnum<visa-resource-name>, "error out"=w357:errorcluster)  [unwired: 11 in]
        n118 = call "RF On_OFF.vi"("VISA Resource Name"=w358, "Status (T:ON)"=w333, "error in (no error)"=w357) -> ("VISA Resource Name Out"=w336:refnum<visa-resource-name>, "error out"=w339:errorcluster)  [unwired: 11 in]
      }
      event "Frequency (MHz)": Value Change {
        n119 = event-data() -> ("NewVal"=w368:dbl)  [unwired: 1 in, 4 out]
        n120 = call "Config Frequency.vi"("VISA Resource Name"=w370, "Freq Offset (0.0)"=0.0, "Freq Multiplier (1.0)"=1.0, "Adjust Phase (0.0)"=0.0, "Frequency (1000.0)"=w368, "Freq Ref (T:ON)"=TRUE, "error in (no error)"=w369, "OptPhNoise (F:MD2 > 10khzOffset)"=FALSE) -> ("VISA Resource Name Out"=w396:refnum<visa-resource-name>, "error out"=w395:errorcluster)  [unwired: 6 in]
        n121 = call "Config Amplitude.vi"("VISA Resource Name"=w396, "Ampl Ref Set (0.00)"=0.0, "Ampl Ref (F:OFF)"=FALSE, "Ampl Offset (0.00)"=0.0, "Amplitude (-135.00)"=w367, "Unit (0:dBm)"=T6."dBm", "Atten Hold (F:OFF)"=FALSE, "error in (no error)"=w395) -> ("VISA Resource Name Out"=w394:refnum<visa-resource-name>, "error out"=w393:errorcluster)  [unwired: 6 in]
        n122 = call "Config FM Modulation.vi"("VISA Resource Name"=w394, "Status (T:ON)"=TRUE, "EXT Source Coupling (F:DC)"=FALSE, "FM Deviation Couple (F:OFF)"=FALSE, "error in (no error)"=w393, "FM Deviation (1.0)"=75.0 ("FM Deviation (75)"), "FM Rate (400.0)"=10000.0 ("FM Rate (10000)"), "FM Waveform (0:SINE)"=T7."SINE") -> ("VISA Resource Name Out"=w392:refnum<visa-resource-name>, "error out"=w391:errorcluster)  [unwired: 10 in]
        n123 = call "ModOn_OFF.vi"("VISA Resource Name"=w392, "Status (T:ON)"=FALSE, "error in (no error)"=w391) -> ("VISA Resource Name Out"=w390:refnum<visa-resource-name>, "error out"=w389:errorcluster)  [unwired: 11 in]
        n124 = call "RF On_OFF.vi"("VISA Resource Name"=w390, "Status (T:ON)"=w366, "error in (no error)"=w389) -> ("VISA Resource Name Out"=w365:refnum<visa-resource-name>, "error out"=w371:errorcluster)  [unwired: 11 in]
      }
    }
  }
  n125 = while "Main Loop" {
    shift-right: [w428] -> w18
    shift-left: w21 -> [w445]
    shift-right: [w439] -> _
    shift-left: _ -> [w444]
    shift-right: [w422] -> _
    shift-left: _ -> [w442]
    shift-right: [w416] -> _
    shift-left: _ -> [w417]
    shift-right: [w399] -> _
    shift-left: _ -> [w414]
    tunnel: w34 -> [w437]
    tunnel: [w430] -> w17
    stop <- w398 stop-if-true
    w415 = FALSE
    n126 = local read "Channel Names"() -> (w402:string[])
    n127 = Wait (ms)(milliseconds to wait=200) -> ()  [unwired: 1 out]
    n128 = local write "Run"(w415) -> ()
    n129 = local write "Running"(w415) -> ()
    n130 = case shown="True" "Compile" {
      tunnel: "Timing File" -> [_ w567]
      tunnel: "Perl Parser" -> [_ w566]
      tunnel: [w563 w568] -> w436
      tunnel: [w564 w569] -> w446
      tunnel: w445 -> [w564 w565]
      tunnel: w444 -> [w563 _]
      frame False {
        n131 = Wait (ms)(milliseconds to wait=10) -> ()  [unwired: 1 out]
      }
      frame True {
        n132 = call "File Parser VI.vi"("error in (no error)"=w565, "Original Timing File Path"=w567, "Perl Parser Path"=w566) -> ("error out"=w569:errorcluster, "Parsed File Path"=w568:path)  [unwired: 7 in]
      }
    }
    "Parsed File Location" <- w436
    n133 = local read "Total Step"() -> (w403:u64)
    n134 = case shown="True" "Load" {
      tunnel: w436 -> [w547 w557]
      tunnel: w446 -> [w548 w561]
      tunnel: [w543 w555] -> w422
      tunnel: [w544 w556] -> w406
      tunnel: [w546 w549] -> w405
      tunnel: [w538 w554] -> w418
      tunnel: [w545 w560] -> w443
      tunnel: [w539 w559] -> w416
      tunnel: [w542 w558] -> w399
      tunnel: [w548 w552] -> w438
      tunnel: [w547 w557] -> w439
      tunnel: "Channel Number (Adjustable)" -> [w546 _]
      tunnel: w402 -> [w545 _]
      tunnel: "Initial States(Adjustable)" -> [w544 _]
      tunnel: w442 -> [w543 _]
      tunnel: w414 -> [w542 _]
      tunnel: w403 -> [w538 _]
      tunnel: [w541 w551] -> w421
      tunnel: "Timing Array (Adjustable)" -> [w541 _]
      tunnel: w417 -> [w539 _]
      tunnel: "Original Timing Signal (adjustable)" -> [w537 _]
      tunnel: [w537 w550] -> w412
      frame False {
        n135 = Wait (ms)(milliseconds to wait=10) -> ()  [unwired: 1 out]
      }
      frame True {
        n136 = call "File Process VI.vi"("error in (no error)"=w561, "Parsed File Path"=w557) -> ("Error Out"=w553:errorcluster, "Total Step"=w554:u64, "Switching Times"=w555:u32[][], "Channel Names"=w560:string[], "Initial States"=w556:u16[], "Channel Number"=w549:u16, "GPIB 1"=w559:string, "GPIB 2"=w558:string)  [unwired: 2 in]
        n137 = call "Timing Process.vi"("Initial States"=w556, "Switching Times"=w555, "Total Steps"=w554, "error in (no error)"=w553, "Channel"=w549) -> ("Output Signal Array"=w550:i16[][], "Output Time Array"=w551:i32[], "error out"=w552:errorcluster)
      }
    }
    "Channel Names" <- w443
    "Total Step" <- w418
    n138 = Quotient & Remainder "#DIO"(x=w405, y=u16 16) -> (floor(x/y)=w404:u16)  [unwired: 1 out]
    n139 = for "Read in Control Signals" {
      N: w404 -> [_]
      tunnel: "DIO Groups" -> [w452] mode=indexing
      tunnel: [w451] -> w410 mode=indexing
      tunnel: [w450] -> w409 mode=indexing
      n140 = call "DataProcess2.vi"("DIO Group 1"=w452) -> ("High"=w451:u16, "Low"=w450:u16)
    }
    n141 = for "Signal Modifier" {
      tunnel: w412 -> [w464] mode=indexing
      tunnel: [w463] -> w423 mode=indexing
      tunnel: w410 -> [w462]
      tunnel: w409 -> [w461]
      tunnel: w404 -> [w460]
      n142 = for {
        N: w460 -> [_]
        tunnel: w464 -> [w469] mode=indexing
        tunnel: [w467] -> w463 mode=indexing
        tunnel: w462 -> [w466] mode=indexing
        tunnel: w461 -> [w465] mode=indexing
        n143 = Or(x=w466, y=w469) -> (x .or. y?=w468:u16)
        n144 = And(x=w468, y=w465) -> (x .and. y?=w467:u16)
      }
    }
    "Modified Timing Signal" <- w423
    n145 = Build Array(w416, w399) -> (→"Quantum Composer Command":string[])
    n146 = local write "Channel Number (Adjustable)"(w405) -> ()
    n147 = local write "Initial States(Adjustable)"(w406) -> ()
    n148 = local write "Original Timing Signal (adjustable)"(w412) -> ()
    n149 = local write "Timing Array (Adjustable)"(w421) -> ()
    n150 = Not(x="All Low") -> (.not. x?=w424:bool)
    n151 = And(x=w424, y="Run") -> (x .and. y?=w425:bool)
    n152 = Initialize Array "LTS"(i16 0, w404) -> (w432:i16[])
    n153 = case shown="True" w425 {
      tunnel: w421 -> [_ w479]
      tunnel: w423 -> [_ w478]
      tunnel: w437 -> [w471 w477]
      tunnel: w438 -> [w470 w476]
      tunnel: "Loop" -> [_ w475]
      tunnel: [w470 w474] -> w429
      tunnel: [w471 w473] -> w431
      tunnel: w404 -> [_ w472]
      frame False {
      }
      frame True {
        n154 = while {
          tunnel: w479 -> [w495]
          tunnel: w478 -> [w494]
          tunnel: w477 -> [w493]
          tunnel: w476 -> [w486]
          tunnel: w475 -> [w483]
          tunnel: [w484] -> w474
          tunnel: [w492] -> w473
          tunnel: w472 -> [w488]
          i -> [w491]
          stop <- w489 continue-if-true
          n155 = for {
            tunnel: w495 -> [w501] mode=indexing
            tunnel: w494 -> [w505] mode=indexing
            tunnel: w493 -> [w508]
            tunnel: w486 -> [w496]
            tunnel: [w507] -> w484
            tunnel: [w504] -> w492
            tunnel: w488 -> [w499]
            w497 = 10  # Time Constant
            n156 = Equal?(x=w501, y=0) -> (x = y?=w502:bool)
            n157 = Greater Or Equal?(x=w501, y=w497) -> (x >= y?=w509:bool)
            n158 = Multiply(x=w501, y=w497) -> (x*y=w500:i32)
            n159 = Quotient & Remainder "#LTS"(x=w501, y=w497) -> (floor(x/y)=w506:i32)  [unwired: 1 out]
            n160 = Quotient & Remainder "#STS"(x=w500, y=w499) -> (floor(x/y)=w498:i32)  [unwired: 1 out]
            n161 = case shown="False" w502 {
              tunnel: w509 -> [w517 _]
              tunnel: w508 -> [w516 w536]
              tunnel: w496 -> [w515 w535]
              tunnel: [w514 w535] -> w507
              tunnel: w506 -> [w513 _]
              tunnel: w505 -> [w512 _]
              tunnel: [w511 w536] -> w504
              tunnel: w498 -> [w510 _]
              frame False {
                n162 = case shown="True" w517 {
                  tunnel: w516 -> [w522 w532]
                  tunnel: w515 -> [w524 w531]
                  tunnel: [w523 w530] -> w514
                  tunnel: w513 -> [_ w529]
                  tunnel: w512 -> [w518 w527]
                  tunnel: [w521 w528] -> w511
                  tunnel: w510 -> [w520 _]
                  frame False {
                    n163 = for {
                      N: w520 -> [_]
                      tunnel: [w525] -> w519 mode=indexing
                      tunnel: w518 -> [w525]
                    }
                    n164 = call-poly <vilib>:"UeiDaqWrite.vi"("error in (no error)"=w524, "Digital Data"=w519, "UeiDaq Refnum In"=w522) -> ("error out"=w523:errorcluster, "UeiDaq Refnum Out"=w521:refnum<k20>)  [unwired: 7 in]
                  }
                  frame True {
                    n165 = Wait (ms)(milliseconds to wait=w529) -> ()  [unwired: 1 out]
                    n166 = for {
                      tunnel: w527 -> [w534] mode=indexing
                      tunnel: [w533] -> w526 mode=indexing
                      n167 = Number To Boolean Array(number=w534) -> (Boolean array=w533:bool[])
                    }
                    "Status Indicator" <- w526
                    n168 = call-poly <vilib>:"UeiDaqWrite.vi"("error in (no error)"=w531, "Digital Data"=w527, "UeiDaq Refnum In"=w532) -> ("error out"=w530:errorcluster, "UeiDaq Refnum Out"=w528:refnum<k20>)  [unwired: 7 in]
                  }
                }
              }
              frame True {
              }
            }
          }
          n169 = Unbundle By Name(w484) -> ("status"=w485:bool)
          n170 = Not(x=w485) -> (.not. x?=w482:bool)
          n171 = And(x=w483, y=w482) -> (x .and. y?=w481:bool)
          n172 = Not(x="stop") -> (.not. x?=w480:bool)
          n173 = And(x=w481, y=w480) -> (x .and. y?=w489:bool)
          "Loop Count" <- w491
          "Running" <- TRUE
        }
      }
    }
    n174 = case shown="True" "Normal Stop" {
      tunnel: w432 -> [_ w459]
      tunnel: w431 -> [w454 w458]
      tunnel: [w454 w457] -> w430
      tunnel: w429 -> [w453 w456]
      tunnel: [w453 w455] -> w428
      frame False {
      }
      frame True {
        n175 = call-poly <vilib>:"UeiDaqWrite.vi"("error in (no error)"=w456, "Digital Data"=w459, "UeiDaq Refnum In"=w458) -> ("error out"=w455:errorcluster, "UeiDaq Refnum Out"=w457:refnum<k20>)  [unwired: 7 in]
      }
    }
    n176 = Or(x="All Low", y="Normal Stop") -> (x .or. y?=w401:bool)
    n177 = Unbundle By Name(w429) -> ("status"=w434:bool)
    n178 = Or(x=w434, y=w401) -> (x .or. y?=w398:bool)
    n179 = property on="Main Loop Stopped?" class="Bool (strict)"("Val(Sgnl)"=w398) -> ()  [unwired: 2 in, 2 out]
  }
  n180 = while "ER Stop Loop" {
    tunnel: w21 -> [w572]
    tunnel: w34 -> [w571]
    tunnel: "DIO Port" -> [w570]
    stop <- w573 stop-if-true
    n181 = event shown="[1] \"All Low\": Value Change" {
      selector: _ -> [_ _ _]
      dyn-events: _ -> [_ _ _]
      timeout: _ -> [_ _ _]
      tunnel: [FALSE w591 w594] -> w573
      tunnel: w572 -> [_ w589 _]
      tunnel: w571 -> [_ w590 _]
      tunnel: w570 -> [_ w575 _]
      event Timeout {
        n182 = event-data() -> ()  [unwired: 1 in, 2 out]
      }
      event "All Low": Value Change {
        w580 = 8  # ALL State cleared regardless of status
        n183 = event-data() -> ("NewVal"=w591:bool)  [unwired: 1 in, 1 out]
        n184 = call <vilib>:"UeiDaqCloseSession.vi"("error in (no error)"=w589, "UeiDaq Refnum In"=w590) -> ("error out"=w576:errorcluster)  [unwired: 8 in, 1 out]
        n185 = local write "Running"(FALSE) -> ()
        n186 = call <vilib>:"UeiDaqShowError.vi"("error in (no error)"=w576) -> ()  [unwired: 10 in, 1 out]
        n187 = call-poly <vilib>:"UeiDaqCreateSession.vi"("error in (no error)"=w576, "Resource"=w575) -> ("error out"=w583:errorcluster, "UeiDaq Refnum Out"=w582:refnum<k20>)  [unwired: 8 in]
        n188 = Initialize Array "LTS"(i16 0, w580) -> (w581:i16[])
        n189 = call-poly <vilib>:"UeiDaqConfigureTiming.vi"("error in (no error)"=w583, "UeiDaq Refnum In"=w582) -> ("error out"=w585:errorcluster, "UeiDaq Refnum Out"=w584:refnum<k20>)  [unwired: 8 in]
        n190 = call-poly <vilib>:"UeiDaqWrite.vi"("error in (no error)"=w585, "Digital Data"=w581, "UeiDaq Refnum In"=w584) -> ("error out"=w578:errorcluster, "UeiDaq Refnum Out"=w577:refnum<k20>)  [unwired: 7 in]
        n191 = call <vilib>:"UeiDaqCloseSession.vi"("error in (no error)"=w578, "UeiDaq Refnum In"=w577) -> ("error out"=w587:errorcluster)  [unwired: 8 in, 1 out]
        n192 = flat-sequence {
          tunnel: [w593] -> w586
          tunnel: w587 -> [w593]
          frame #0 {
            w592 = FALSE
            n193 = local write "Loop"(w592) -> ()
            n194 = local write "Running"(w592) -> ()
            n195 = local write "All Low"(w592) -> ()
            n196 = local write "Run"(w592) -> ()
          }
        }
        n197 = call <vilib>:"UeiDaqShowError.vi"("error in (no error)"=w586) -> ()  [unwired: 10 in, 1 out]
      }
      event "Normal Stop": Value Change {
        n198 = event-data() -> ("NewVal"=w594:bool)  [unwired: 1 in, 3 out]
      }
    }
  }
  n199 = call <vilib>:"ULx Clear Task.vi"("task in"=w24, "error in"=w23) -> ("error out"=w30:errorcluster)  [unwired: 13 in]
  n200 = call <vilib>:"Simple Error Handler.vi"("type of dialog (OK msg:1)"=w28, "error in (no error)"=w30) -> ()  [unwired: 3 in, 5 out]
  n201 = call "Error Query.vi"("VISA Resource Name"=w2, "error in (no error)"=w9) -> ("VISA Resource Name Out"=w11:refnum<visa-resource-name>, "error out"=w14:errorcluster)  [unwired: 10 in, 2 out]
  n202 = call "Error Message.vi"("VISA Resource Name"=w11, "error in (no error)"=w14) -> ("VISA Resource Name Out"=w12:refnum<visa-resource-name>, "error out"=w13:errorcluster)  [unwired: 9 in, 3 out]
  n203 = call "Close.vi"("VISA Resource Name"=w12, "error in (no error)"=w13) -> ("error out"=→"error out":errorcluster)  [unwired: 13 in]
  n204 = call <vilib>:"UeiDaqCloseSession.vi"("error in (no error)"=w18, "UeiDaq Refnum In"=w17) -> ("error out"=w16:errorcluster)  [unwired: 8 in, 1 out]
  n205 = call <vilib>:"UeiDaqShowError.vi"("error in (no error)"=w16) -> ()  [unwired: 10 in, 1 out]
